vi "Save_to_Project.vi"(8 "error in (no error)":errorcluster, 9 "index":string, 10 "buildObject":T1, 11 "niLabel in":refnum<class "niLabel.lvclass">) -> (0 "error out":errorcluster, 1 "index out":string, 2 "buildObject out":T1, 3 "niLabel out":refnum<class "niLabel.lvclass">, 5 "saved?":bool)   [LabVIEW 2020, in "niLabel.lvclass"]
uses:
  <vilib>/AppBuilder/IB_Classes/Destination/niLabel/niLabel.lvclass
  <vilib>/AppBuilder/IB_Classes/Destination/niLabel/niLabel.lvclass/niLabel.ctl
  <resource>/Framework/Providers/API/ItemRef.ctl
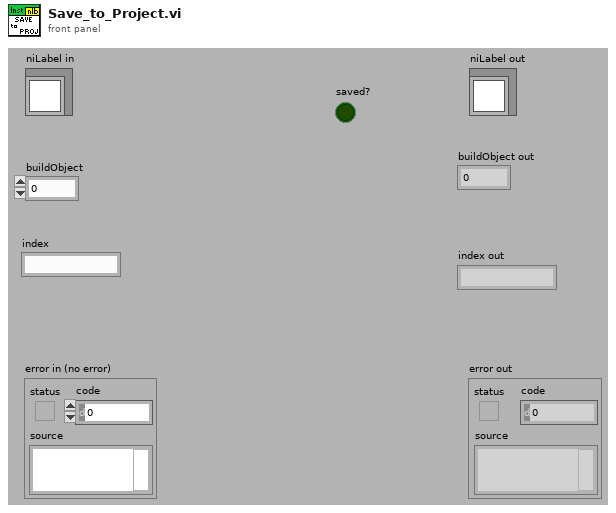
[diagram p1: front panel]
types:
  T1 = typedef "ItemRef.ctl" = u64
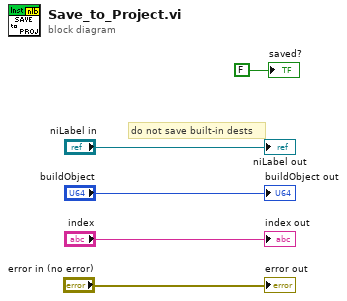
[diagram p0: block diagram]
diagram:
  # "do not save built-in dests"
  "error out" <- "error in (no error)"
  "niLabel out" <- "niLabel in"
  "index out" <- "index"
  "buildObject out" <- "buildObject"
  "saved?" <- FALSE ("saved?")
